vi "Bertta_v07_1.vi"() -> ()   [LabVIEW 2015]
panel:
  in  "OK Button":bool
  in  "Tab Control":T1(tab)
  in  "Description":string
  in  "Project name":string
  in  "User (initials)":string
  out "PUMP 1":bool
  out "Target amount":dbl
  out "Scale weight":dbl
  out "Amount now":dbl
  out "Flow rate":dbl
  out "Time to target":dbl format="%<%H:%M:%S>t"
  out "Current step":dbl
  out "Target amount":dbl
  out "Amount now":dbl
  out "Tr":dbl
  out "Tj in":dbl
  out "Tj out":dbl
  out "T init":dbl
  out "T set":dbl
  out "Current step":i32
  out "RPM":dbl
  out "Torque 2":dbl
  out "Waveform Chart 5":dynamicdata(graph)
  out "Waveform Chart 6":dynamicdata(graph)
  out "Waveform Chart 7":dynamicdata(graph)
  in  "Tab Control 2":T2(tab)
  out "Waveform Chart 3":dynamicdata(graph)
  out "Waveform Chart 8":dynamicdata(graph)
  out "Waveform Chart 9":dynamicdata(graph)
  out "Table":string[][](table)
  in  "Headers":string[](array[string])=["Flow rate, P1, g/min", "Weight, S1, g", "Amount / step, P1, g", "Step Number, P1", "Total amount, P1, g", "Tj in, C", "Tj out, C", "Tr, C", "RPM", "Torque"]
  out "Boolean 12":bool
  out "Boolean 7":bool
  out "Boolean 6":bool
  out "Boolean 5":bool
  out "Boolean 4":bool
  in  "?":bool
  in  "Tbypass":dbl=20.0
  in  "Tfail":dbl=22.0
  in  "err":i32
  in  "Lauda port":dbl=9.0
  out "Data out":dbl
  in  "Bypass select":enum32{"Tr", "Tj"}(radio)
  in  "Seq":dbl[][](array[numeric])=[[20.0, 45.0, 50.0], [46.0, 50.0, 20.0], [3.0, 3.0, 3.0]]
  out "T control":dbl
  out "Tr":dbl
  out "Tj in":dbl
  out "Tj out":dbl
  out "DT":dbl
  out "Elapsed":i32
  out "Current step":i32
  in  "PAUSE":bool
  out "Tinit":dbl
  out "Tset":dbl
  out "Time limit":dbl
  out "Waveform Chart":dynamicdata(graph)
  out "Data out":dbl
  in  "Port":i32=10
  in  "Radio Buttons":enum32{"Reglo Digital", "Reglo Analog", "PAM"}(radio)
  out "Speed":dbl
  out "mA":dbl format="%#_2g"
  in  "Port":i32=15
  out "RPM":dbl format="%#_2g"
  out "Boolean 18":bool
  out "Boolean 17":bool
  out "Boolean 16":bool
  out "Boolean 15":bool
  out "Boolean 14":bool
  out "Boolean 13":bool
  out "Boolean 11":bool
  out "Boolean 10":bool
  out "Boolean 9":bool
  out "Boolean 8":bool
  in  "Seq 2":dbl[][](array[numeric])=[[3.0, 3.0, 7.0], [2.0, 2.0, 2.0], [4.0, 2.0, 100.0]]
  in  "?":bool
  out "Flow rate (g/min)":dbl
  out "Time (min)":dbl
  out "Target (g)":dbl
  out "Scale reading":dbl
  out "Step amount now":dbl
  out "Time to target":dbl format="%<%H:%M:%S>t"
  in  "Bypass (g/min)":dbl
  out "Waveform Chart 2":dynamicdata(graph)
  in  "?":bool
  out "Total amount now":dbl
  out "Total time":dbl
  out "Total amount target":dbl
  out "RPM":dbl
  out "Torque":dbl
  in  "Set RPM":dbl(slide) scale=0.0..500.0
  out "Waveform Chart 4":dynamicdata(graph)
  in  "?":T3(tab)
  in  "Device port":dbl=13.0
  # "PUMP & SCALE 1"
  # "STEP"
  # "TOTAL"
  # "Tinit     >    Tset       min. time"
  # "Grams    /   min"
  # "Pump configuration"
  # "Scale configuration"
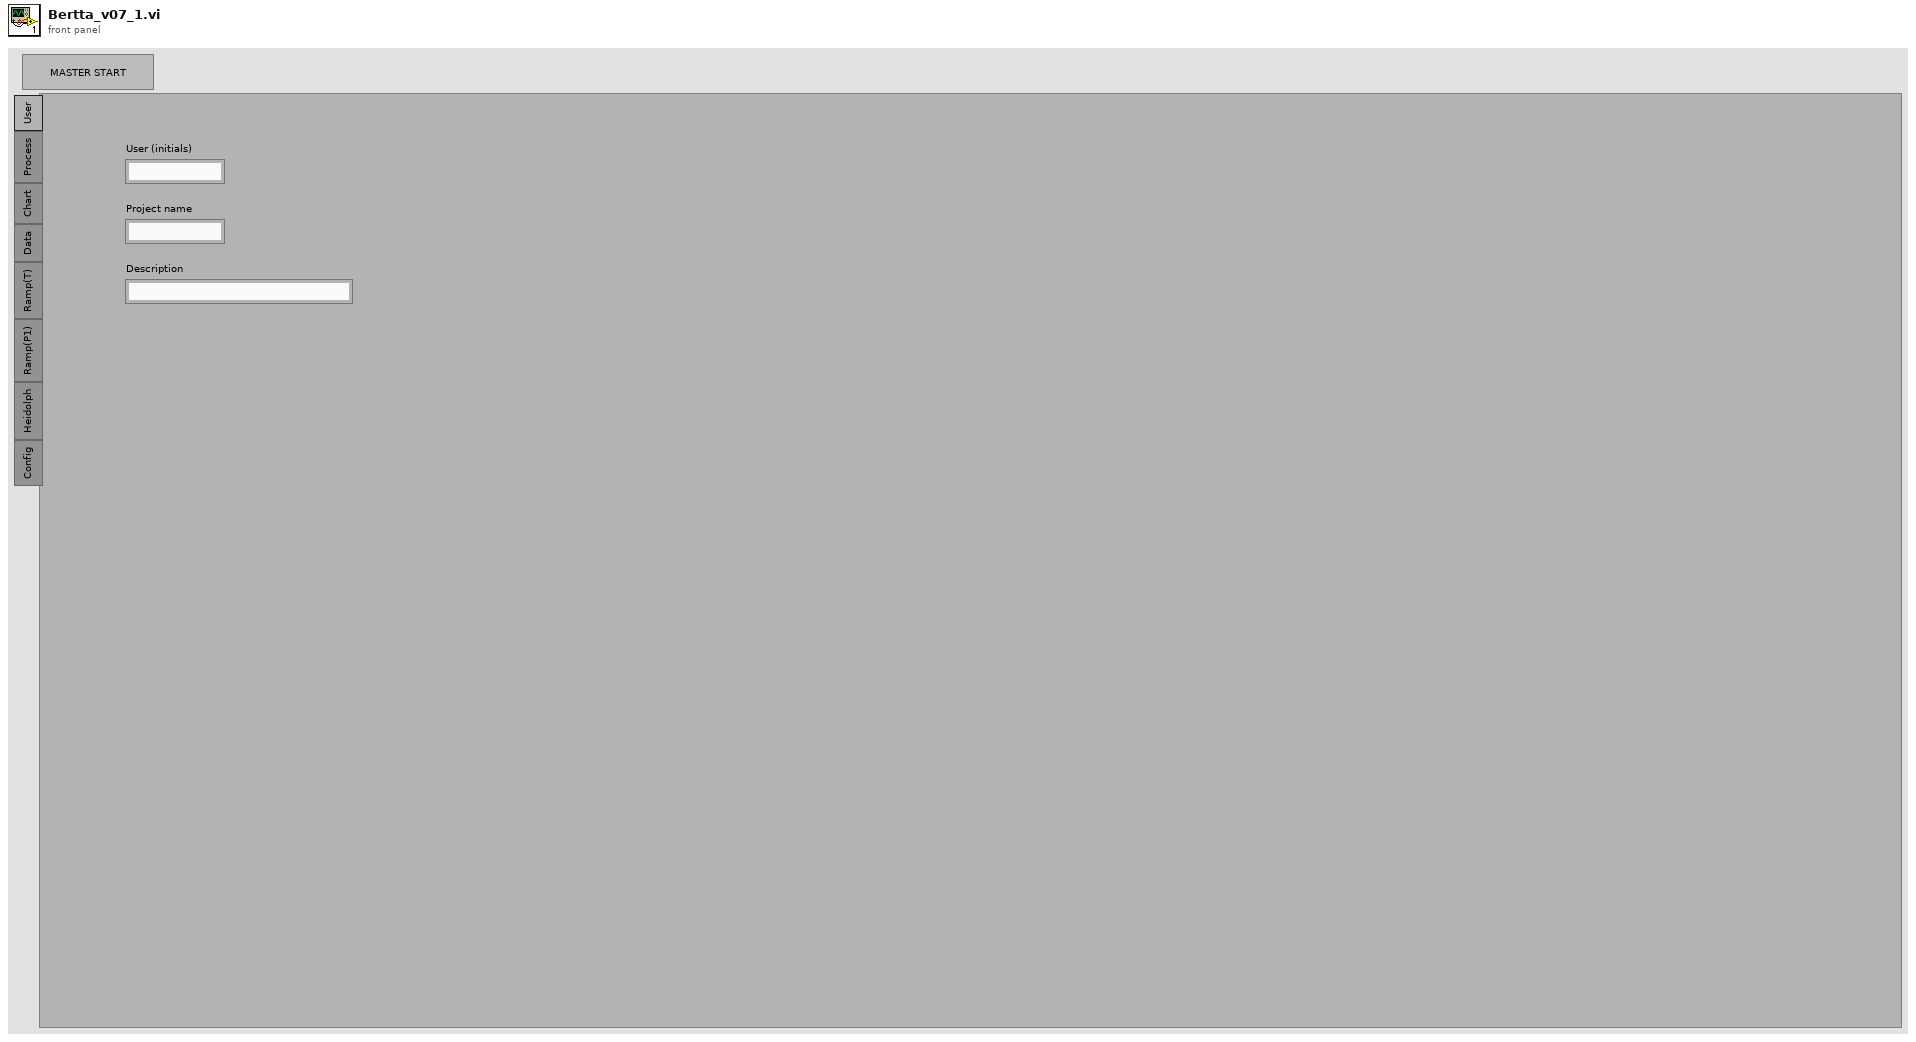
[diagram p1: front panel]
types:
  T1 = enum32{"User", "Process", "Chart", "Data", "Ramp(T)", "Ramp(P1)", "Heidolph", "Config"}
  T2 = enum32{"Temperatures", "Scale / Pump 1", "RPM / torque"}
  T3 = enum32{"DB / File", "Lauda", "Heidolph", "Mettler 1", "Mettler 2", "Mettler 3", "Ismatec 1"}
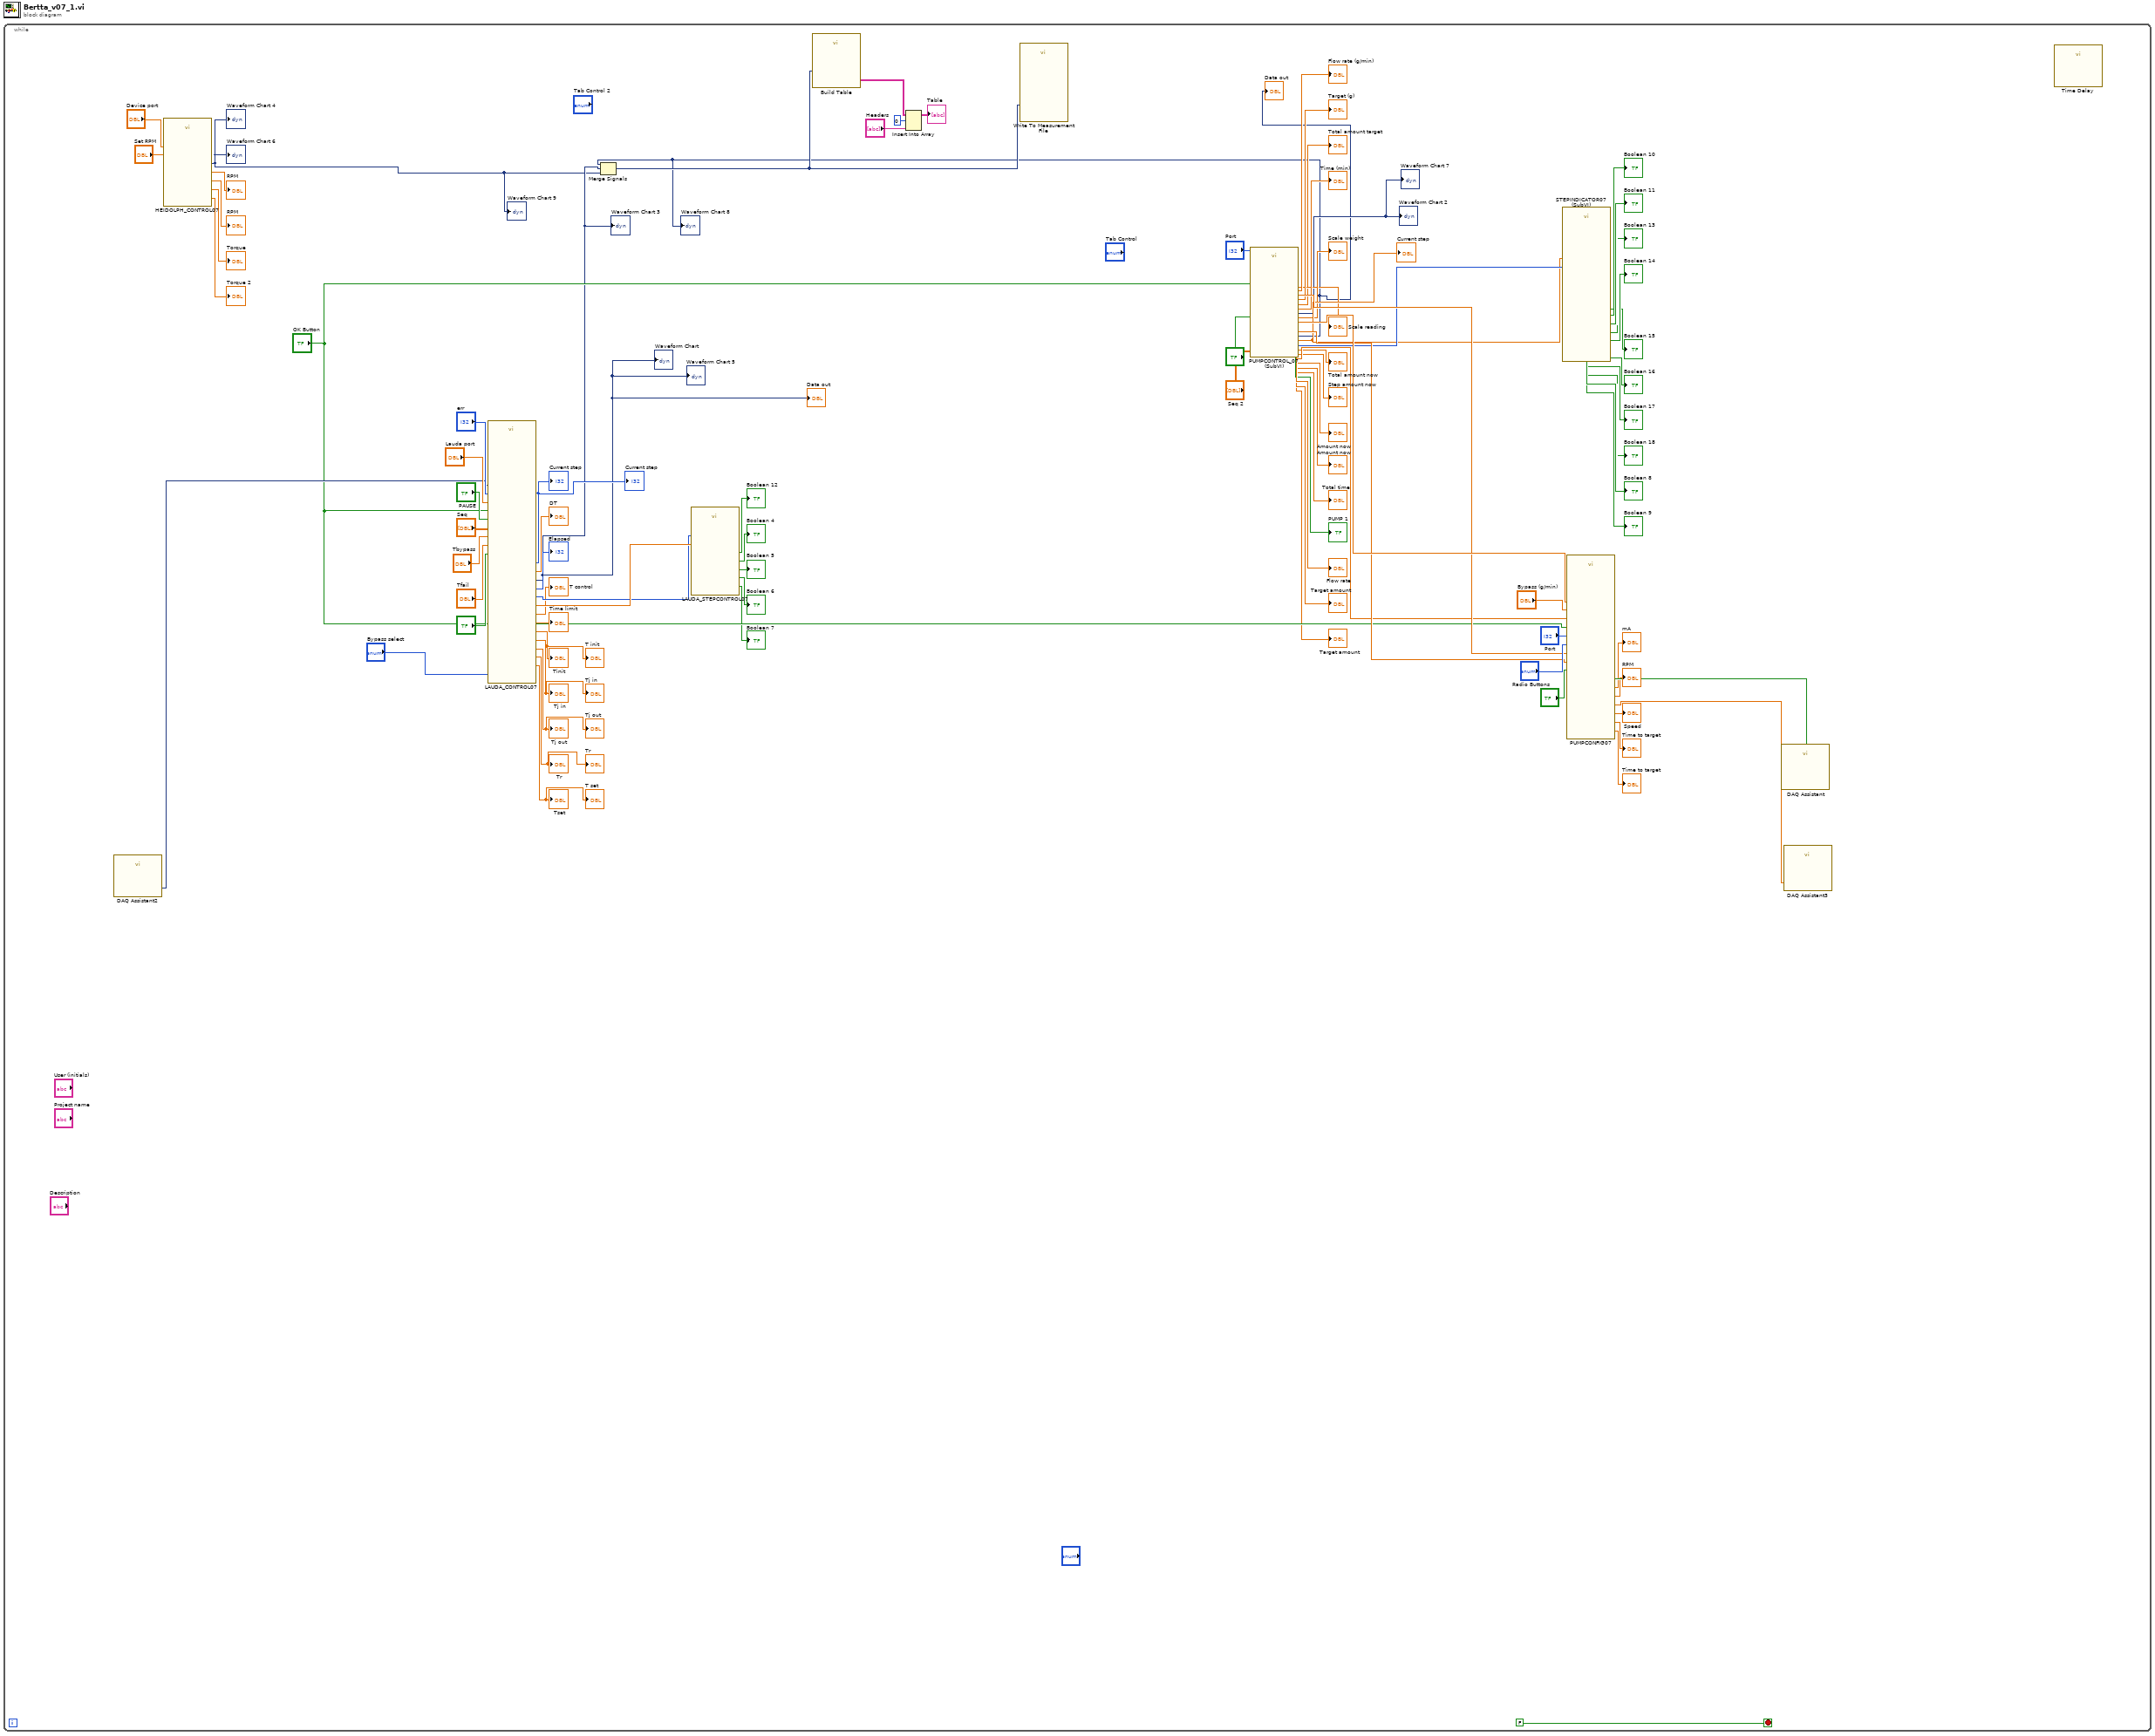
[diagram p0: block diagram]
diagram:
  n1 = while {
    stop <- FALSE stop-if-true
    n2 = call "DAQ Assistant2"() -> ("data"=w67:dynamicdata)  [unwired: 17 in, 2 out]
    n3 = call "HEIDOLPH_CONTROL07.vi"("Set RPM"="Set RPM", "Device port"="Device port") -> ("Dynamic Data"=w6:dynamicdata, "RPM"=→"RPM":dbl, "RPM 2"=→"RPM":dbl, "Torque"=→"Torque":dbl, "Torque 2"=→"Torque 2":dbl)  [unwired: 5 in]
    "Waveform Chart 4" <- w6
    "Waveform Chart 6" <- w6
    "Waveform Chart 9" <- w6
    n4 = call "LAUDA_CONTROL07.vi"(0:"?", "PAUSE"="PAUSE", "data"=w67, "Seq"="Seq", "Lauda port"="Lauda port", "Tbypass"="Tbypass", "Tfail"="Tfail", "Bypass select"="Bypass select", "err"="err", "OK Button"="OK Button") -> (12:"Tj out"=→"Tj in" →"Tj in":dbl, "DT"=→"DT":dbl, 16:"Tj out"=→"Tj out" →"Tj out":dbl, "Tset"=→"Tset" →"T set":dbl, "Dynamic Data"=w8:dynamicdata, "Time limit"=→"Time limit":dbl, "Numeric"=w74:i16, "Numeric 2"=w75:dbl, "T control"=→"T control":dbl, "Current step"=→"Current step" →"Current step":i32, "Elapsed"=→"Elapsed":i32, "Tr"=→"Tr" →"Tr":dbl, "Tinit"=→"Tinit" →"T init":dbl)  [unwired: 5 in]
    "Waveform Chart 3" <- w8
    "Waveform Chart" <- w8
    "Data out" <- w8
    "Waveform Chart 5" <- w8
    n5 = call "LAUDA_STEPCONTROL07.vi"("Numeric 2"=w75, "Numeric"=w74) -> ("Boolean 6"=→"Boolean 6":bool, "Boolean 5"=→"Boolean 5":bool, "Boolean 4"=→"Boolean 4":bool, "Boolean 7"=→"Boolean 7":bool, "Boolean 12"=→"Boolean 12":bool)  [unwired: 5 in]
    n6 = call "PUMPCONTROL_07 (SubVI).vi"("Port"="Port", "OK Button"="OK Button", 2:"?", "Seq in"="Seq 2") -> ("Amount now"=→"Amount now":dbl, "Amount now 2"=→"Amount now":dbl, "Flow rate out"=w57:dbl, "Step amount now"=→"Step amount now":dbl, "Total amount now"=→"Total amount now":dbl, "Total time"=→"Total time":dbl, "Numeric 2"=w63:i16, "PUMP 1"=→"PUMP 1":bool, "Numeric"=w56:dbl, "Flow rate"=→"Flow rate":dbl, "Dynamic Data"=w7:dynamicdata, "Target amount"=→"Target amount":dbl, "Time (min) 2"=w64:dbl, "Target amount 2"=→"Target amount":dbl, "Scale reading"=→"Scale reading":dbl, "Flow rate (g/min)"=→"Flow rate (g/min)":dbl, "Target (g) 2"=w65:dbl, "Target (g)"=→"Target (g)":dbl, "Total amount target"=→"Total amount target":dbl, "Time (min)"=→"Time (min)":dbl, "Waveform Chart 2"=→"Waveform Chart 2" →"Waveform Chart 7":dynamicdata, "Scale weight"=→"Scale weight":dbl, "Amount (g)"=w66:dbl)  [unwired: 1 in]
    "Current step" <- w56
    "Data out" <- w7
    "Waveform Chart 8" <- w7
    n7 = Merge Signals(w7, w8, w6) -> (w9:dynamicdata)
    n8 = call "Build Table"("Signals"=w9) -> ("Table"=w84:string[][])  [unwired: 4 in, 6 out]
    n9 = Insert Into Array(array=w84, index (row)=0, new element="Headers") -> (→"Table":string[][])  [unwired: 1 in]
    n10 = call "Write To Measurement File"("Signals"=w9) -> ()  [unwired: 16 in, 3 out]
    n11 = call "STEPINDICATOR07 (SubVI).vi"("Numeric"=w56, "Numeric 2"=w63) -> ("Boolean 18"=→"Boolean 18":bool, "Boolean 8"=→"Boolean 8":bool, "Boolean 9"=→"Boolean 9":bool, "Boolean 17"=→"Boolean 17":bool, "Boolean 10"=→"Boolean 10":bool, "Boolean 16"=→"Boolean 16":bool, "Boolean 11"=→"Boolean 11":bool, "Boolean 15"=→"Boolean 15":bool, "Boolean 14"=→"Boolean 14":bool, "Boolean 13"=→"Boolean 13":bool)  [unwired: 4 in]
    n12 = call "PUMPCONFIG07.vi"(0:"?", "Radio Buttons"="Radio Buttons", "Bypass (g/min)"="Bypass (g/min)", "Target (g) in"=w65, "Amount (g)"=w66, "Time (min) in"=w64, "Flow rate in"=w57, "OK Button"="OK Button", "Port"="Port") -> ("Time to target 2"=→"Time to target":dbl, "Time to target"=→"Time to target":dbl, "mA"=→"mA":dbl, "signal"=w72:dbl, "Speed"=→"Speed":dbl, "RPM"=→"RPM":dbl, "Array"=w73:bool[])
    n13 = call "DAQ Assistant"("data"=w73) -> ()  [unwired: 17 in, 2 out]
    n14 = call "DAQ Assistant3"("data"=w72) -> ()  [unwired: 17 in, 2 out]
    n15 = call "Time Delay"() -> ()  [unwired: 11 in, 1 out]
  }
